vi "CRYSet Analysis Editor Front Panel.vi"(11 "Vi Ref":refnum<vi>) -> ()   [LabVIEW 2013]
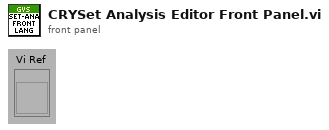
[diagram p1: front panel]
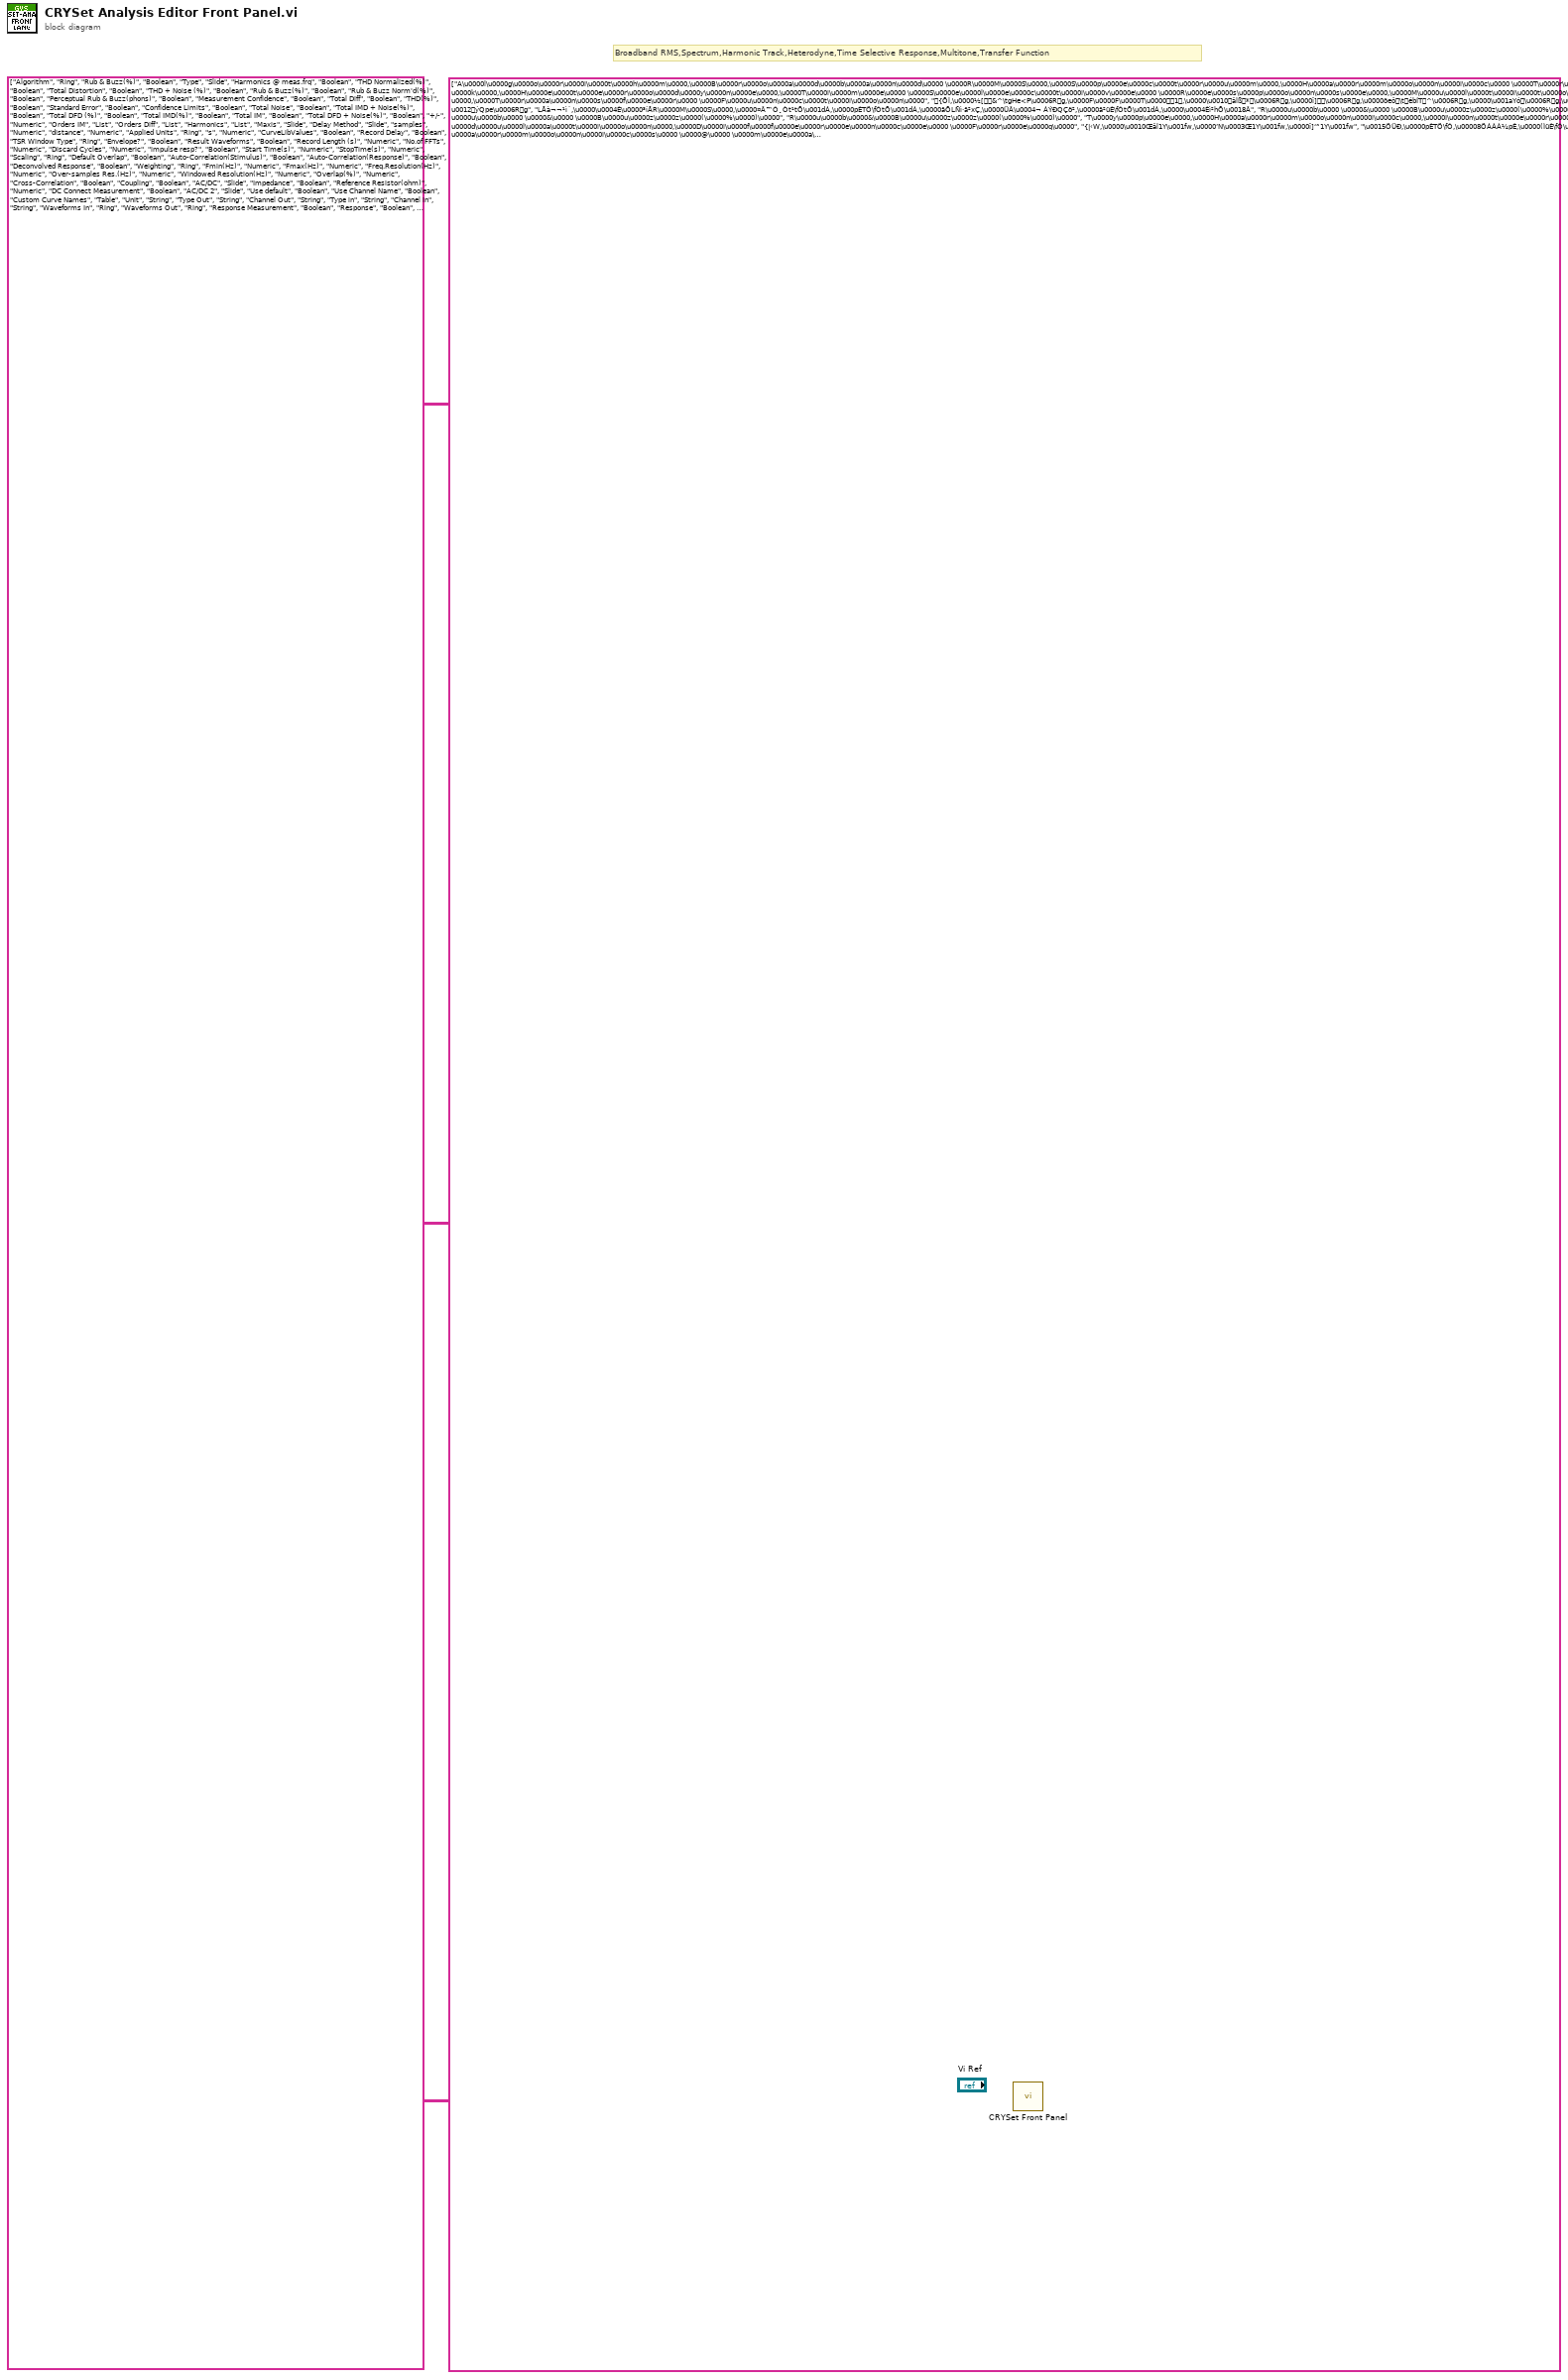
[diagram p0: block diagram]
diagram:
  # "Broadband RMS,Spectrum,Harmonic Track,Heterodyne,Time Selective Response,Multitone,Transfer Function"
  # "Caption, Tab Page, Multilist Header, Button 4"
  # "Control Type"
  # "Control Name and Tab"
  n1 = call "CRYSet Front Panel.vi"("Caption(Boolean Text)"=string[][] [["A\u0000l\u0000g\u0000o\u0000r\u0000i\u0000t\u0000h\u0000m\u0000,\u0000B\u0000r\u0000o\u0000a\u0000d\u0000b\u0000a\u0000n\u0000d\u0000 \u0000R\u0000M\u0000S\u0000,\u0000S\u0000p\u0000e\u0000c\u0000t\u0000r\u0000u\u0000m\u0000,\u0000H\u0000a\u0000r\u0000m\u0000o\u0000n\u0000i\u0000c\u0000 \u0000T\u0000r\u0000a\u0000c\u0000k\u0000,\u0000H\u0000e\u0000t\u0000e\u0000r\u0000o\u0000d\u0000y\u0000n\u0000e\u0000,\u0000T\u0000i\u0000m\u0000e\u0000 \u0000S\u0000e\u0000l\u0000e\u0000c\u0000t\u0000i\u0000v\u0000e\u0000 \u0000R\u0000e\u0000s\u0000p\u0000o\u0000n\u0000s\u0000e\u0000,\u0000M\u0000u\u0000l\u0000t\u0000i\u0000t\u0000o\u0000n\u0000e\u0000,\u0000T\u0000r\u0000a\u0000n\u0000s\u0000f\u0000e\u0000r\u0000 \u0000F\u0000u\u0000n\u0000c\u0000t\u0000i\u0000o\u0000n\u0000", "{Õl,\u0000½[&^\tgHe<P\u0006Rg,\u0000F\u0000F\u0000T\u00001,\u0000\u0010âlß*\u0006Rg,\u0000î]\u0006Rg,\u0000öeô\tébÍT^\u0006Rg,\u0000\u001aYó\u0006Rg,\u0000 O\u0012ýQpe\u0006Rg", "LÅà¬¬¹ì´,\u0000\u0004È\u0000³íÅR\u0000M\u0000S\u0000,\u0000¤Â™Ó¸Òt¹tÕ\u001dÁ,\u0000pÈTÖ\fÓtÕ\u001dÁ,\u0000äÕLÑì·ä²xÇ,\u0000ÜÂ\u0004¬ ÁÝÐQÇõ²,\u0000ä²üÈ\fÓtÕ\u001dÁ,\u0000\u0004Èì²hÕ\u0018Â"], ["R\u0000u\u0000b\u0000 \u0000&\u0000 \u0000B\u0000u\u0000z\u0000z\u0000(\u0000%\u0000)\u0000", "R\u0000u\u0000b\u0000 \u0000&\u0000 \u0000B\u0000u\u0000z\u0000z\u0000(\u0000%\u0000)\u0000", "R\u0000u\u0000b\u0000&\u0000B\u0000u\u0000z\u0000z\u0000(\u0000%\u0000)\u0000"], ["T\u0000y\u0000p\u0000e\u0000,\u0000H\u0000a\u0000r\u0000m\u0000o\u0000n\u0000i\u0000c\u0000,\u0000I\u0000n\u0000t\u0000e\u0000r\u0000m\u0000o\u0000d\u0000u\u0000l\u0000a\u0000t\u0000i\u0000o\u0000n\u0000,\u0000D\u0000i\u0000f\u0000f\u0000e\u0000r\u0000e\u0000n\u0000c\u0000e\u0000 \u0000F\u0000r\u0000e\u0000q\u0000", "{|‹W,\u0000\u0010Œâl1Y\u001fw,\u0000’N\u0003Œ1Y\u001fw,\u0000î]‘˜1Y\u001fw", "\u0015ÖÜÐ,\u0000pÈTÖ\fÓ,\u00008ÖÁÀÀ¼pÈ,\u0000(ÌüÈ\fÓ\u0018Â"], ["H\u0000a\u0000r\u0000m\u0000o\u0000n\u0000i\u0000c\u0000s\u0000 \u0000@\u0000 \u0000m\u0000e\u0000a\u0000s\u0000.\u0000f\u0000r\u0000q\u0000", "\u0010ŒâlKmÏ‘‘˜‡s", "pÈTÖ\fÓ!Î\u0015ÈüÈ\fÓ\u0018Â"], ["T\u0000H\u0000D\u0000 \u0000N\u0000o\u0000r\u0000m\u0000a\u0000l\u0000i\u0000z\u0000e\u0000d\u0000(\u0000%\u0000)\u0000", ";`\u0010Œâl1Y\u001fw(\u0000R_\u0000N\u0016S)\u0000(\u0000%\u0000)\u0000", "T\u0000H\u0000D\u0000\u0015ÈÜ­TÖ(\u0000%\u0000)\u0000"], ["T\u0000o\u0000t\u0000a\u0000l\u0000 \u0000D\u0000i\u0000s\u0000t\u0000o\u0000r\u0000t\u0000i\u0000o\u0000n\u0000", ";`1Y\u001fw", "\u0004È´ÌtÇÀÉì·ÐÉ"], ["T\u0000H\u0000D\u0000 \u0000+\u0000 \u0000N\u0000o\u0000i\u0000s\u0000e\u0000 \u0000(\u0000%\u0000)\u0000", ";`\u0010Œâl1Y\u001fw+\u0000jVðX(\u0000%\u0000)\u0000", "T\u0000H\u0000D\u0000+\u0000¡ÇLÇ(\u0000%\u0000)\u0000"], ["R\u0000u\u0000b\u0000 \u0000&\u0000 \u0000B\u0000u\u0000z\u0000z\u0000(\u0000%\u0000)\u0000", "\u0002_ó—", "R\u0000u\u0000b\u0000 \u0000&\u0000 \u0000B\u0000u\u0000z\u0000z\u0000(\u0000%\u0000)\u0000"], ["R\u0000u\u0000b\u0000 \u0000&\u0000 \u0000B\u0000u\u0000z\u0000z\u0000 \u0000N\u0000o\u0000r\u0000m\u0000'\u0000d\u0000(\u0000%\u0000)\u0000", "\u0002_ó—(\u0000R_\u0000N\u0016S)\u0000(\u0000%\u0000)\u0000", "R\u0000u\u0000b\u0000&\u0000B\u0000u\u0000z\u0000z\u0000\u0015ÈÜ­TÖ(\u0000%\u0000)\u0000"], ["P\u0000e\u0000r\u0000c\u0000e\u0000p\u0000t\u0000u\u0000a\u0000l\u0000 \u0000R\u0000u\u0000b\u0000 \u0000&\u0000 \u0000B\u0000u\u0000z\u0000z\u0000(\u0000p\u0000h\u0000o\u0000n\u0000s\u0000)\u0000", "\u001faåw\u0002_ó—(\u0000p\u0000h\u0000o\u0000n\u0000s\u0000)\u0000", "ÀÉ\u0001¬ \u0000R\u0000u\u0000b\u0000 \u0000&\u0000 \u0000B\u0000u\u0000z\u0000z\u0000(\u0000p\u0000h\u0000o\u0000n\u0000s\u0000)\u0000"], ["M\u0000e\u0000a\u0000s\u0000u\u0000r\u0000e\u0000m\u0000e\u0000n\u0000t\u0000 \u0000C\u0000o\u0000n\u0000f\u0000i\u0000d\u0000e\u0000n\u0000c\u0000e\u0000", "KmÏ‘náO¦^", "ÿ»LÇ1Á!Î\u0015È"], ["T\u0000o\u0000t\u0000a\u0000l\u0000 \u0000D\u0000i\u0000f\u0000f\u0000", ";`î]\u0002_", "\u0004È´Ì \u0000(ÌtÇÀÉì·ÐÉ"], ["T\u0000H\u0000D\u0000(\u0000%\u0000)\u0000", ";`\u0010Œâl1Y\u001fw(\u0000%\u0000)\u0000", "T\u0000H\u0000D\u0000(\u0000%\u0000)\u0000"], ["S\u0000t\u0000a\u0000n\u0000d\u0000a\u0000r\u0000d\u0000 \u0000E\u0000r\u0000r\u0000o\u0000r\u0000", "\u0007hÆQî]", "\\Ô\u0000É$Æ(Ì"], ["C\u0000o\u0000n\u0000f\u0000i\u0000d\u0000e\u0000n\u0000c\u0000e\u0000 \u0000L\u0000i\u0000m\u0000i\u0000t\u0000s\u0000", "náOLuP–", "ÿ»LÇ1Á\\ÕÄ¬"], ["T\u0000o\u0000t\u0000a\u0000l\u0000 \u0000N\u0000o\u0000i\u0000s\u0000e\u0000", ";`jVðX", "\u0004È´Ì¡ÇLÇ"], ["T\u0000o\u0000t\u0000a\u0000l\u0000 \u0000I\u0000M\u0000D\u0000 \u0000+\u0000 \u0000N\u0000o\u0000i\u0000s\u0000e\u0000(\u0000%\u0000)\u0000", "qQ\tgI\u0000M\u0000D\u0000+\u0000jVðX(\u0000%\u0000)\u0000", "\u0004È´Ì \u0000I\u0000M\u0000D\u0000+\u0000¡ÇLÇ(\u0000%\u0000)\u0000"], ["T\u0000o\u0000t\u0000a\u0000l\u0000 \u0000D\u0000F\u0000D\u0000 \u0000(\u0000%\u0000)\u0000", "qQ\tgD\u0000F\u0000D\u0000(\u0000%\u0000)\u0000", "\u0004È´Ì \u0000D\u0000F\u0000D\u0000 \u0000(\u0000%\u0000)\u0000"], ["T\u0000o\u0000t\u0000a\u0000l\u0000 \u0000I\u0000M\u0000D\u0000(\u0000%\u0000)\u0000", "qQ\tgI\u0000M\u0000D\u0000(\u0000%\u0000)\u0000", "\u0004È´Ì \u0000I\u0000M\u0000D\u0000(\u0000%\u0000)\u0000"], ["T\u0000o\u0000t\u0000a\u0000l\u0000 \u0000I\u0000M\u0000", "qQ\tgI\u0000M\u0000", "\u0004È´Ì \u0000I\u0000M\u0000tÇÀÉì·ÐÉ"], ["T\u0000o\u0000t\u0000a\u0000l\u0000 \u0000D\u0000F\u0000D\u0000 \u0000+\u0000 \u0000N\u0000o\u0000i\u0000s\u0000e\u0000(\u0000%\u0000)\u0000", "qQ\tgD\u0000F\u0000D\u0000+\u0000jVðX(\u0000%\u0000)\u0000", "\u0004È´Ì \u0000D\u0000F\u0000D\u0000+\u0000¡ÇLÇ(\u0000%\u0000)\u0000"], ["S\u0000t\u0000d\u0000 \u0000E\u0000r\u0000r\u0000", "\u0007hÆQ\u0019•ï‹", "\\Ô\u0000É$Æ(Ì"], ["O\u0000r\u0000d\u0000e\u0000r\u0000s\u0000", "!kpe", "(Ì\u0018Â"], ["O\u0000r\u0000d\u0000e\u0000r\u0000s\u0000", "!kpe", "(Ì\u0018Â"], ["H\u0000a\u0000r\u0000m\u0000o\u0000n\u0000i\u0000c\u0000s\u0000", "\u0010Œâl", "pÈTÖ\fÓ"], ["M\u0000a\u0000x\u0000i\u0000s\u0000,\u0000x\u0000,\u0000y\u0000,\u0000z\u0000", "t,\u0000x\u0000,\u0000y\u0000,\u0000z\u0000", "Ç¬¹\\ÔÍ,\u0000x\u0000,\u0000y\u0000,\u0000z\u0000"], ["D\u0000e\u0000l\u0000a\u0000y\u0000 \u0000M\u0000e\u0000t\u0000h\u0000o\u0000d\u0000,\u0000A\u0000u\u0000t\u0000o\u0000 \u0000D\u0000e\u0000l\u0000a\u0000y\u0000,\u0000S\u0000e\u0000t\u0000 \u0000V\u0000a\u0000l\u0000u\u0000e\u0000s\u0000,\u0000C\u0000u\u0000r\u0000v\u0000e\u0000s\u0000 \u0000L\u0000i\u0000b\u0000r\u0000a\u0000r\u0000y\u0000", "ö^ß¹eÕl,\u0000ê¨Rö^öe,\u0000¾[<P,\u0000òf¿~^", "ÀÉðÅ)¼¼,\u0000ÇÙ³ÀÉðÅ,\u0000\u0012¬$Á\u0015È,\u0000á¬ Á\u001cÁà¬¬¹©Æ"], ["s\u0000a\u0000m\u0000p\u0000l\u0000e\u0000s\u0000", "7h,g", "\\Ôø¼\u001c¬\u0018Â"], ["d\u0000i\u0000s\u0000t\u0000a\u0000n\u0000c\u0000e\u0000", "Ý»y", "p¬¬¹"], ["A\u0000p\u0000p\u0000l\u0000i\u0000e\u0000d\u0000 \u0000U\u0000n\u0000i\u0000t\u0000s\u0000", "”^(uUSMO", "\u0001È©Æè²\u0004Ç"], ["s\u0000", "Òy", "\bÍ"], ["C\u0000u\u0000r\u0000v\u0000e\u0000L\u0000i\u0000b\u0000r\u0000a\u0000r\u0000y\u0000V\u0000a\u0000l\u0000u\u0000e\u0000s\u0000", "òf¿~<P", "á¬ Á\u001cÁà¬\u0012¬"], ["R\u0000e\u0000c\u0000o\u0000r\u0000d\u0000 \u0000D\u0000e\u0000l\u0000a\u0000y\u0000", "°U_ö^ß", "0®]¸ÀÉðÅ"], ["T\u0000S\u0000R\u0000 \u0000W\u0000i\u0000n\u0000d\u0000o\u0000w\u0000 \u0000T\u0000y\u0000p\u0000e\u0000", "T\u0000S\u0000R\u0000—zýQpe{|‹W", "T\u0000S\u0000R\u0000=ÌhÕ\u0018Â"], ["T\u0000i\u0000m\u0000e\u0000 \u0000E\u0000n\u0000v\u0000e\u0000l\u0000o\u0000p\u0000e\u0000", "öeô•\u0005SÜ~", "ÜÂ\u0004¬ìÓ}·"], ["R\u0000e\u0000s\u0000u\u0000l\u0000t\u0000 \u0000W\u0000a\u0000v\u0000e\u0000f\u0000o\u0000r\u0000m\u0000s\u0000", "Ó~œgâlb_", "°¬ü¬\fÓ\u0015Ö"], ["R\u0000e\u0000c\u0000o\u0000r\u0000d\u0000 \u0000L\u0000e\u0000n\u0000g\u0000t\u0000h\u0000 \u0000(\u0000s\u0000)\u0000", "F\u0000F\u0000T\u0000•¦^(\u0000s\u0000)\u0000", "0®]¸8®tÇ(\u0000\bÍ)\u0000"], ["N\u0000o\u0000.\u0000o\u0000f\u0000 \u0000F\u0000F\u0000T\u0000s\u0000", "F\u0000F\u0000T\u0000peϑ", "F\u0000F\u0000T\u0000\u0014¾\\¸lÐ\u001c¬\u0018Â"], ["D\u0000i\u0000s\u0000c\u0000a\u0000r\u0000d\u0000 \u0000C\u0000y\u0000c\u0000l\u0000e\u0000s\u0000", "\"N\u0003_hT\u001fg", "„¼¼¹üÈ0®"], ["I\u0000m\u0000p\u0000u\u0000l\u0000s\u0000e\u0000 \u0000R\u0000e\u0000s\u0000p\u0000.\u0000", "²QûQÍT”^", "„Ç\fÕ¤ÂQÇõ²"], ["S\u0000t\u0000a\u0000r\u0000t\u0000 \u0000T\u0000i\u0000m\u0000e\u0000(\u0000s\u0000)\u0000", "\u0000_ËYöeô•(\u0000Òy)\u0000", "ÜÂ‘ÇÜÂ\u0004¬(\u0000\bÍ)\u0000"], ["S\u0000t\u0000o\u0000p\u0000 \u0000T\u0000i\u0000m\u0000e\u0000(\u0000s\u0000)\u0000", "\\Pbköeô•(\u0000Òy)\u0000", "\u0015ÈÀÉÜÂ\u0004¬(\u0000\bÍ)\u0000"], ["S\u0000c\u0000a\u0000l\u0000i\u0000n\u0000g\u0000", ";R¦^", "™ÌÄ³"], ["D\u0000e\u0000f\u0000a\u0000u\u0000l\u0000t\u0000 \u0000O\u0000v\u0000e\u0000r\u0000l\u0000a\u0000p\u0000", "Øž¤‹Í‘àS", "0®\u0015È¹¬hÎ"], ["A\u0000u\u0000t\u0000o\u0000-\u0000C\u0000o\u0000r\u0000r\u0000e\u0000l\u0000a\u0000t\u0000i\u0000o\u0000n\u0000(\u0000S\u0000t\u0000i\u0000m\u0000u\u0000l\u0000u\u0000s\u0000)\u0000", "ê¨RøvsQ(\u0000Ào±R)\u0000", "ÇÙ³ÁÀ\u0000­(\u0000Çù­)\u0000"], ["A\u0000u\u0000t\u0000o\u0000-\u0000C\u0000o\u0000r\u0000r\u0000e\u0000l\u0000a\u0000t\u0000i\u0000o\u0000n\u0000(\u0000R\u0000e\u0000s\u0000p\u0000o\u0000n\u0000s\u0000e\u0000)\u0000", "ê¨RøvsQ(\u0000ÍT^)\u0000", "ÇÙ³ÁÀ\u0000­(\u0000QÇõ²)\u0000"], ["D\u0000e\u0000c\u0000o\u0000n\u0000v\u0000o\u0000l\u0000v\u0000e\u0000d\u0000 \u0000R\u0000e\u0000s\u0000p\u0000o\u0000n\u0000s\u0000e\u0000", "\u0006wSïyÍT^", "íÅ\u0011É©ÌQÇõ²"], ["W\u0000e\u0000i\u0000g\u0000h\u0000t\u0000i\u0000n\u0000g\u0000", " RCg", "4»Œ¬"], ["F\u0000m\u0000i\u0000n\u0000(\u0000H\u0000z\u0000)\u0000", "\u0000gNO‘˜‡s(\u0000H\u0000z\u0000)\u0000", "\\ÍŒÁüÈ\fÓ\u0018Â(\u0000H\u0000z\u0000)\u0000"], ["F\u0000m\u0000a\u0000x\u0000(\u0000H\u0000z\u0000)\u0000", "\u0000g'Y‘˜‡s(\u0000H\u0000z\u0000)\u0000", "\\Í\u0000³üÈ\fÓ\u0018Â(\u0000H\u0000z\u0000)\u0000"], ["F\u0000r\u0000e\u0000q\u0000.\u0000R\u0000e\u0000s\u0000o\u0000l\u0000u\u0000t\u0000i\u0000o\u0000n\u0000(\u0000H\u0000z\u0000)\u0000", "‘˜‡sÍT”^(\u0000H\u0000z\u0000)\u0000", "üÈ\fÓ\u0018Â„½tÕ¥²(\u0000H\u0000z\u0000)\u0000"], ["O\u0000v\u0000e\u0000r\u0000-\u0000s\u0000a\u0000m\u0000p\u0000l\u0000e\u0000s\u0000 \u0000R\u0000e\u0000s\u0000.\u0000(\u0000H\u0000z\u0000)\u0000", "òf¿~\u0006R¨s(\u0000H\u0000z\u0000)\u0000", "\u0004È´Ì\\Ôø¼„½tÕ¥²(\u0000H\u0000z\u0000)\u0000"], ["W\u0000i\u0000n\u0000d\u0000o\u0000w\u0000e\u0000d\u0000 \u0000R\u0000e\u0000s\u0000o\u0000l\u0000u\u0000t\u0000i\u0000o\u0000n\u0000(\u0000H\u0000z\u0000)\u0000", "zýQpe\u0006R¨s(\u0000H\u0000z\u0000)\u0000", "=Ì„½tÕ¥²(\u0000H\u0000z\u0000)\u0000"], ["O\u0000v\u0000e\u0000r\u0000l\u0000a\u0000p\u0000(\u0000%\u0000)\u0000", "Í‘àS(\u0000%\u0000)\u0000", "¹¬hÎ(\u0000%\u0000)\u0000"], ["C\u0000r\u0000o\u0000s\u0000s\u0000-\u0000C\u0000o\u0000r\u0000r\u0000e\u0000l\u0000a\u0000t\u0000i\u0000o\u0000n\u0000", "’NøvsQ", "8ÖÁÀÁÀ\u0000­"], ["C\u0000o\u0000u\u0000p\u0000l\u0000i\u0000n\u0000g\u0000", "&€\bT", "°¬iÕ"], ["A\u0000C\u0000/\u0000D\u0000C\u0000,\u0000A\u0000C\u0000,\u0000D\u0000C\u0000", "A\u0000C\u0000/\u0000D\u0000C\u0000,\u0000¤NAm,\u0000ôvAm", "P­X¹/\u0000ÁÉX¹,\u0000P­X¹,\u0000ÁÉX¹"], ["I\u0000m\u0000p\u0000e\u0000d\u0000a\u0000n\u0000c\u0000e\u0000", ";–—b", "DÆ\u0004È\u0000ÈmÕ"], ["R\u0000e\u0000f\u0000e\u0000r\u0000e\u0000n\u0000c\u0000e\u0000 \u0000R\u0000e\u0000s\u0000i\u0000s\u0000t\u0000o\u0000r\u0000(\u0000o\u0000h\u0000m\u0000)\u0000", "ÂS\u0003€5u;–(\u0000o\u0000h\u0000m\u0000)\u0000", "8Ìà¬\u0000ÈmÕ(\u0000o\u0000h\u0000m\u0000)\u0000"], ["D\u0000C\u0000 \u0000C\u0000o\u0000n\u0000n\u0000e\u0000c\u0000t\u0000 \u0000M\u0000e\u0000a\u0000s\u0000u\u0000r\u0000e\u0000m\u0000e\u0000n\u0000t\u0000", "D\u0000C\u0000Þ¥cKmÏ", "ÁÉX¹(¸°¬!Î\u0015È"], ["A\u0000C\u0000/\u0000D\u0000C\u0000 \u00002\u0000,\u0000A\u0000(\u0000 \u0000i\u0000n\u0000 \u0000V\u0000o\u0000l\u0000t\u0000a\u0000g\u0000e\u0000 \u0000s\u0000o\u0000u\u0000r\u0000c\u0000e\u0000 \u0000M\u0000o\u0000d\u0000e\u0000)\u0000,\u0000V\u0000(\u0000 \u0000i\u0000n\u0000 \u0000C\u0000u\u0000r\u0000r\u0000e\u0000n\u0000t\u0000 \u0000s\u0000o\u0000u\u0000r\u0000c\u0000e\u0000 \u0000M\u0000o\u0000d\u0000e\u0000)\u0000", "A\u0000C\u0000/\u0000D\u0000C\u0000 \u00002\u0000,\u0000A\u0000(\u00005uSn!j\u000f_)\u0000,\u0000V\u0000(\u0000(W5uAmn!j\u000f_)\u0000", "P­X¹/\u0000ÁÉX¹,\u0000TÅ˜ÓDÅ(\u0000\u0004ÈUÅÐÆœÌ)¼ÝÂ)\u0000,\u0000ü¼¸Ò(\u0000\u0004ÈX¹ÐÆœÌ)¼ÝÂ)\u0000"], ["U\u0000s\u0000e\u0000 \u0000d\u0000e\u0000f\u0000a\u0000u\u0000l\u0000t\u0000", "O(uØž¤‹", "0®\u0015È¬À©Æ"], ["U\u0000s\u0000e\u0000 \u0000C\u0000h\u0000a\u0000n\u0000n\u0000e\u0000l\u0000 \u0000N\u0000a\u0000m\u0000e\u0000", "O(uS\rTðy", "µÑ\\¸tÇ„¹¬À©Æ"], ["C\u0000u\u0000s\u0000t\u0000o\u0000m\u0000 \u0000C\u0000u\u0000r\u0000v\u0000e\u0000 \u0000N\u0000a\u0000m\u0000e\u0000s\u0000", "ê[INvòf¿~\rTðy", "á¬ ÁtÇ„¹\u0015ÈXÇ"], ["U\u0000n\u0000i\u0000t\u0000", "USMO", "è²\u0004Ç"], ["T\u0000y\u0000p\u0000e\u0000 \u0000O\u0000u\u0000t\u0000", "úQ{|W", "œÍl­\u0015ÖÜÐ"], ["C\u0000h\u0000a\u0000n\u0000n\u0000e\u0000l\u0000 \u0000O\u0000u\u0000t\u0000", "úQ\u001aS", "œÍl­µÑ\\¸"], ["T\u0000y\u0000p\u0000e\u0000 \u0000i\u0000n\u0000", "eQ{|W", "…Çl­\u0015ÖÜÐ"], ["C\u0000h\u0000a\u0000n\u0000n\u0000e\u0000l\u0000 \u0000i\u0000n\u0000", "eQ\u001aS", "…Çl­µÑ\\¸"], ["W\u0000a\u0000v\u0000e\u0000f\u0000o\u0000r\u0000m\u0000s\u0000 \u0000I\u0000n\u0000", "eQâlb_", "…Çl­\fÓ\u0015Ö"], ["W\u0000a\u0000v\u0000e\u0000f\u0000o\u0000r\u0000m\u0000s\u0000 \u0000O\u0000u\u0000t\u0000", "úQâlb_", "œÍl­\fÓ\u0015Ö"], ["R\u0000e\u0000s\u0000p\u0000o\u0000n\u0000s\u0000e\u0000 \u0000M\u0000e\u0000a\u0000s\u0000u\u0000r\u0000e\u0000m\u0000e\u0000n\u0000t\u0000", "ÍT”^KmÏ‘", "QÇõ²!Î\u0015È"], ["R\u0000e\u0000s\u0000p\u0000o\u0000n\u0000s\u0000e\u0000", "ÍT”^", "QÇõ²"], ["S\u0000t\u0000i\u0000m\u0000u\u0000l\u0000u\u0000s\u0000", "Ào±R", "Çù­"], ["R\u0000e\u0000s\u0000p\u0000o\u0000n\u0000s\u0000e\u0000 \u0000M\u0000e\u0000a\u0000s\u0000u\u0000r\u0000e\u0000m\u0000e\u0000n\u0000t\u00001\u0000,\u0000A\u0000b\u0000s\u0000o\u0000l\u0000u\u0000t\u0000e\u0000,\u0000R\u0000e\u0000l\u0000a\u0000t\u0000i\u0000v\u0000e\u0000", "‘˜ÍTKmÏ‘<P,\u0000Ý~ù[<P,\u0000øvù[<P", "QÇõ²!Î\u0015È,\u0000\bÈ\u0000³,\u0000ÁÀ\u0000³"], ["A\u0000p\u0000p\u0000l\u0000y\u0000 \u0000C\u0000o\u0000r\u0000r\u0000e\u0000c\u0000t\u0000i\u0000o\u0000n\u0000 \u0000O\u0000u\u0000t\u0000", "^(uúQîOck", "œÍl­ô¼\u0015È\u0001È©Æ"], ["A\u0000p\u0000p\u0000l\u0000y\u0000 \u0000C\u0000o\u0000r\u0000r\u0000e\u0000c\u0000t\u0000i\u0000o\u0000n\u0000 \u0000i\u0000n\u0000", "^(ueQîOck", "…Çl­ô¼\u0015È\u0001È©Æ"], ["A\u0000v\u0000e\u0000r\u0000a\u0000g\u0000i\u0000n\u0000g\u0000", "s^GW", "ÉÓà­"], ["F\u0000u\u0000n\u0000c\u0000t\u0000i\u0000o\u0000n\u0000s\u0000", "ŸRý€", "0®¥²"], ["S\u0000p\u0000e\u0000c\u0000t\u0000r\u0000a\u0000l\u0000 \u0000S\u0000c\u0000a\u0000l\u0000i\u0000n\u0000g\u0000*\u0000,\u0000R\u0000M\u0000S\u0000,\u0000S\u0000p\u0000e\u0000c\u0000t\u0000r\u0000a\u0000l\u0000 \u0000D\u0000e\u0000n\u0000s\u0000i\u0000t\u0000y\u0000", "‘˜1Œ)>e*\u0000,\u0000\tgHe<P,\u0000‘˜1ŒÆ[¦^", "¤Â™Ó¸Òt¹™ÌÄ³,\u0000R\u0000M\u0000S\u0000,\u0000S\u0000p\u0000e\u0000c\u0000t\u0000r\u0000a\u0000l\u0000 \u0000D\u0000e\u0000n\u0000s\u0000i\u0000t\u0000y\u0000"], ["A\u0000u\u0000t\u0000o\u0000-\u0000S\u0000p\u0000e\u0000c\u0000t\u0000r\u0000u\u0000m\u0000(\u0000S\u0000t\u0000i\u0000m\u0000u\u0000l\u0000u\u0000s\u0000)\u0000*\u0000", "ê¨R1(\u0000Ào±R)\u0000", "ÇÙ³¤ÂÓ¸Òt¹(\u0000Çù­)\u0000"], ["A\u0000u\u0000t\u0000o\u0000-\u0000S\u0000p\u0000e\u0000c\u0000t\u0000r\u0000u\u0000m\u0000(\u0000R\u0000e\u0000s\u0000p\u0000o\u0000n\u0000s\u0000e\u0000)\u0000*\u0000", "ê¨R1(\u0000ÍT^)\u0000", "ÇÙ³¤ÂÓ¸Òt¹(\u0000QÇõ²)\u0000"], ["C\u0000r\u0000o\u0000s\u0000s\u0000-\u0000S\u0000p\u0000e\u0000c\u0000t\u0000r\u0000u\u0000m\u0000*\u0000", "¤NÉS‘˜1Œ*\u0000", "P­(Ì¤Â™Ó¸Òt¹"], ["C\u0000o\u0000h\u0000e\u0000r\u0000e\u0000n\u0000t\u0000 \u0000P\u0000o\u0000w\u0000e\u0000r\u0000*\u0000", "øvr^ŸR‡s*\u0000", "\u0004¬-Á\u0004È%¸"], ["F\u0000r\u0000e\u0000q\u0000u\u0000e\u0000n\u0000c\u0000y\u0000 \u0000R\u0000e\u0000s\u0000p\u0000o\u0000n\u0000s\u0000e\u0000", "‘˜‡sÍT”^", "üÈ\fÓ\u0018ÂQÇõ²"], ["N\u0000o\u0000n\u0000-\u0000C\u0000o\u0000h\u0000e\u0000r\u0000e\u0000n\u0000t\u0000 \u0000P\u0000o\u0000w\u0000e\u0000r\u0000*\u0000", "^—øvr^ŸR‡s*\u0000", "D¾\u0004¬-Á\u0004È%¸"], ["C\u0000o\u0000h\u0000e\u0000r\u0000e\u0000n\u0000c\u0000e\u0000 \u0000(\u0000%\u0000)\u0000", "øvr^(\u0000%\u0000)\u0000", "\u0004¬-Á1Á(\u0000%\u0000)\u0000"], ["N\u0000o\u0000n\u0000-\u0000C\u0000o\u0000h\u0000e\u0000r\u0000e\u0000n\u0000c\u0000e\u0000 \u0000(\u0000%\u0000)\u0000", "^—øvr^(\u0000%\u0000)\u0000", "D¾\u0004¬-Á1Á(\u0000%\u0000)\u0000"], ["S\u0000i\u0000g\u0000n\u0000a\u0000l\u0000-\u0000N\u0000o\u0000i\u0000s\u0000e\u0000 \u0000R\u0000a\u0000t\u0000i\u0000o\u0000 \u0000(\u0000d\u0000B\u0000)\u0000", "áOjVÔk(\u0000d\u0000B\u0000)\u0000", "àÂ8Ö\u0000³¡ÇLÇD¾(\u0000%\u0000)\u0000"], ["N\u0000o\u0000n\u0000-\u0000C\u0000o\u0000h\u0000e\u0000r\u0000e\u0000n\u0000t\u0000 \u0000D\u0000i\u0000s\u0000t\u0000o\u0000r\u0000t\u0000i\u0000o\u0000n\u0000*\u0000", "^—øvr^1Y\u001fw", "D¾\u0004¬-ÁtÇÀÉì·ÐÉ"], ["A\u0000v\u0000e\u0000r\u0000a\u0000g\u0000i\u0000n\u0000g\u00001\u0000,\u0000C\u0000o\u0000m\u0000p\u0000l\u0000e\u0000x\u0000,\u0000P\u0000o\u0000w\u0000e\u0000r\u0000", "s^GW,\u0000\rY\bT,\u0000ŸR‡s", "ÉÓà­,\u0000õ¼ŒÁ,\u0000\u0004È%¸"], ["L\u0000o\u0000o\u0000s\u0000e\u0000 \u0000P\u0000a\u0000r\u0000t\u0000i\u0000c\u0000l\u0000e\u0000", "~gce»yP[", "Ç Ç½¹Ç"], ["L\u0000o\u0000o\u0000s\u0000e\u0000 \u0000P\u0000a\u0000r\u0000t\u0000i\u0000c\u0000l\u0000e\u0000 \u0000W\u0000a\u0000v\u0000e\u0000f\u0000o\u0000r\u0000m\u0000", "~gce»yP[âlb_", "Ç Ç½¹Ç\fÓ\u0015Ö"], ["A\u0000v\u0000e\u0000r\u0000a\u0000g\u0000i\u0000n\u0000g\u0000 \u0000T\u0000i\u0000m\u0000e\u0000(\u0000s\u0000)\u0000", "s^GWöeô•(\u0000s\u0000)\u0000", "ÉÓà­ÜÂ\u0004¬(\u0000\bÍ)\u0000"], ["A\u0000t\u0000t\u0000a\u0000c\u0000k\u0000 \u0000T\u0000h\u0000r\u0000e\u0000s\u0000h\u0000o\u0000l\u0000d\u0000(\u0000d\u0000B\u0000)\u0000", "ÀoÑSLuP–(\u0000d\u0000B\u0000)\u0000", "õ¬©¬1Ñ\u0012¬(\u0000d\u0000B\u0000)\u0000"], ["M\u0000a\u0000x\u0000 \u0000d\u0000u\u0000r\u0000a\u0000t\u0000i\u0000o\u0000n\u0000(\u0000s\u0000)\u0000", "\u0000g'Y\u0001cí~öeô•(\u0000s\u0000)\u0000", "\\Í\u0000³ÀÉÁÜÂ\u0004¬(\u0000\bÍ)\u0000"], ["M\u0000i\u0000n\u0000 \u0000d\u0000u\u0000r\u0000a\u0000t\u0000i\u0000o\u0000n\u0000(\u0000s\u0000)\u0000", "\u0000g\u000f\\\u0001cí~öeô•(\u0000s\u0000)\u0000", "\\ÍÁÀÉÁÜÂ\u0004¬(\u0000\bÍ)\u0000"], ["H\u0000y\u0000s\u0000t\u0000e\u0000r\u0000e\u0000s\u0000i\u0000s\u0000 \u0000U\u0000p\u0000(\u0000d\u0000B\u0000)\u0000", "ÁxÞn°saŒ\nNGS(\u0000d\u0000B\u0000)\u0000", "ÃÆÇ0®¬¹%¸(\u0000d\u0000B\u0000)\u0000"], ["A\u0000p\u0000p\u0000l\u0000y\u0000", "”^(u", "\u0001È©Æ"], ["U\u0000n\u0000i\u0000t\u0000s\u0000.\u0000.\u0000.\u0000", "USMO", "è²\u0004Ç$Á\u0015È"], ["E\u0000d\u0000i\u0000t\u0000 \u0000L\u0000i\u0000s\u0000t\u0000", "\u0016\u0017Rh", "¸ÓÑÉ©º]¸"], ["C\u0000u\u0000r\u0000v\u0000e\u0000s\u0000,\u0000D\u0000e\u0000l\u0000a\u0000y\u0000,\u0000F\u0000r\u0000e\u0000q\u0000u\u0000e\u0000n\u0000c\u0000y\u0000,\u0000L\u0000o\u0000o\u0000s\u0000e\u0000 \u0000P\u0000a\u0000r\u0000t\u0000,\u0000W\u0000a\u0000v\u0000e\u0000f\u0000o\u0000r\u0000m\u0000s\u0000,\u0000D\u0000i\u0000s\u0000t\u0000o\u0000r\u0000t\u0000i\u0000o\u0000n\u0000,\u0000T\u0000i\u0000m\u0000e\u0000,\u0000E\u0000e\u0000l\u0000e\u0000c\u0000t\u0000r\u0000i\u0000c\u0000a\u0000l\u0000,\u0000H\u0000e\u0000l\u0000p\u0000", "òf¿~,\u0000ö^ß,\u0000s,\u0000~gce»yP[,\u0000âlb_,\u00001Y\u001fw,\u0000öeô,\u00005uáO÷S,\u0000.^©R", "Íl­á¬ Á,\u0000ÀÉðÅ,\u0000üÈ\fÓ\u0018Â,\u0000Ç Ç½¹Ç,\u0000ÜÂ\u0004¬\fÓ\u0015Ö,\u0000tÇÀÉì·ÐÉ,\u0000ÜÂ\u0004¬,\u0000\u0004È0®,\u0000Ä³ÀÆÐ¹"], ["A\u0000d\u0000v\u0000a\u0000n\u0000c\u0000e\u0000d\u0000 \u0000V\u0000i\u0000e\u0000w\u0000", "Ø§~\ty", "Ç8Á× \u0000ô¼0®"], ["M\u0000e\u0000t\u0000h\u0000o\u0000d\u0000,\u0000I\u0000E\u0000C\u0000 \u0000M\u0000e\u0000t\u0000h\u0000o\u0000d\u0000,\u0000I\u0000E\u0000E\u0000E\u0000 \u0000M\u0000e\u0000t\u0000h\u0000o\u0000d\u0000", "¹eÕl,\u0000I\u0000E\u0000C\u0000¹eÕl,\u0000I\u0000E\u0000E\u0000E\u0000¹eÕl", ")¼•¼,\u0000I\u0000E\u0000C\u0000 \u0000)¼•¼,\u0000I\u0000E\u0000E\u0000E\u0000 \u0000)¼•¼"], ["I\u0000m\u0000p\u0000e\u0000d\u0000a\u0000n\u0000c\u0000e\u0000", ";–—b", "DÆ\u0004È\u0000ÈmÕ"], ["S\u0000p\u0000e\u0000c\u0000t\u0000r\u0000a\u0000", "‘˜1Œ", "¤Â™Ó¸Òt¹"], ["D\u0000i\u0000s\u0000t\u0000a\u0000n\u0000c\u0000e\u0000 \u0000U\u0000n\u0000i\u0000t\u0000,\u0000i\u0000n\u0000c\u0000h\u0000e\u0000s\u0000,\u0000m\u0000e\u0000t\u0000e\u0000r\u0000s\u0000", "Ý»yUSMO,\u0000ñø[,\u0000s|", "D\u0000i\u0000s\u0000t\u0000a\u0000n\u0000c\u0000e\u0000 \u0000U\u0000n\u0000i\u0000t\u0000,\u0000i\u0000n\u0000c\u0000h\u0000e\u0000s\u0000,\u0000m\u0000e\u0000t\u0000e\u0000r\u0000s\u0000"], ["C\u0000u\u0000r\u0000v\u0000e\u0000 \u0000R\u0000e\u0000s\u0000o\u0000l\u0000u\u0000t\u0000i\u0000o\u0000n\u0000", "òf¿~\u0006R¨", "á¬ Á„½tÕ¥²"], ["P\u0000o\u0000l\u0000a\u0000r\u0000i\u0000t\u0000y\u0000", "g'`", "ù­1Á"], ["I\u0000m\u0000p\u0000e\u0000d\u0000a\u0000n\u0000c\u0000e\u0000", ";–—b", "„Ç<ÕX³¤Â"], ["A\u0000m\u0000p\u0000 \u0000A\u0000u\u0000t\u0000o\u0000 \u0000M\u0000o\u0000d\u0000e\u0000,\u0000A\u0000u\u0000t\u0000o\u0000m\u0000a\u0000t\u0000i\u0000c\u0000,\u0000M\u0000a\u0000n\u0000u\u0000a\u0000l\u0000", "L\u0000a\u0000n\u0000g\u0000u\u0000a\u0000g\u0000e\u0000 \u0000M\u0000o\u0000d\u0000e\u0000,\u0000ê¨R,\u0000Kb¨R", "L\u0000a\u0000n\u0000g\u0000u\u0000a\u0000g\u0000e\u0000 \u0000M\u0000o\u0000d\u0000e\u0000,\u0000ÇÙ³,\u0000\u0018ÂÙ³"], ["M\u0000i\u0000c\u0000r\u0000o\u0000p\u0000h\u0000o\u0000n\u0000e\u0000", "¦žKQÎ˜", "È¹tÇlÐ"], ["M\u0000i\u0000c\u0000 \u0000R\u0000e\u0000s\u0000i\u0000s\u0000t\u0000o\u0000r\u0000(\u0000o\u0000h\u0000m\u0000)\u0000", "¦žKQÎ˜5u;–(\u0000o\u0000h\u0000m\u0000)\u0000", "È¹tÇlÐ\u0000ÈmÕ(\u0000o\u0000h\u0000m\u0000)\u0000"], ["A\u0000m\u0000p\u0000 \u0000A\u0000u\u0000t\u0000o\u0000 \u0000M\u0000o\u0000d\u0000e\u0000,\u0000A\u0000u\u0000t\u0000o\u0000m\u0000a\u0000t\u0000i\u0000c\u0000,\u0000M\u0000a\u0000n\u0000u\u0000a\u0000l\u0000", "L\u0000a\u0000n\u0000g\u0000u\u0000a\u0000g\u0000e\u0000 \u0000M\u0000o\u0000d\u0000e\u0000,\u0000ê¨R,\u0000Kb¨R", "L\u0000a\u0000n\u0000g\u0000u\u0000a\u0000g\u0000e\u0000 \u0000M\u0000o\u0000d\u0000e\u0000,\u0000ÇÙ³,\u0000\u0018ÂÙ³"], ["M\u0000i\u0000c\u0000 \u0000C\u0000u\u0000r\u0000r\u0000e\u0000n\u0000t\u0000", "¦žKQÎ˜5uAm", "È¹tÇlÐ\u0004ÈX¹"]], "Control ID and Type(Label Name, Type)"=string[][] [["Algorithm", "Ring"], ["Rub & Buzz(%)", "Boolean"], ["Type", "Slide"], ["Harmonics @ meas.frq", "Boolean"], ["THD Normalized(%)", "Boolean"], ["Total Distortion", "Boolean"], ["THD + Noise (%)", "Boolean"], ["Rub & Buzz(%)", "Boolean"], ["Rub & Buzz Norm'd(%)", "Boolean"], ["Perceptual Rub & Buzz(phons)", "Boolean"], ["Measurement Confidence", "Boolean"], ["Total Diff", "Boolean"], ["THD(%)", "Boolean"], ["Standard Error", "Boolean"], ["Confidence Limits", "Boolean"], ["Total Noise", "Boolean"], ["Total IMD + Noise(%)", "Boolean"], ["Total DFD (%)", "Boolean"], ["Total IMD(%)", "Boolean"], ["Total IM", "Boolean"], ["Total DFD + Noise(%)", "Boolean"], ["+/-", "Numeric"], ["Orders IM", "List"], ["Orders Diff", "List"], ["Harmonics", "List"], ["Maxis", "Slide"], ["Delay Method", "Slide"], ["samples", "Numeric"], ["distance", "Numeric"], ["Applied Units", "Ring"], ["s", "Numeric"], ["CurveLibValues", "Boolean"], ["Record Delay", "Boolean"], ["TSR Window Type", "Ring"], ["Envelope?", "Boolean"], ["Result Waveforms", "Boolean"], ["Record Length (s)", "Numeric"], ["No.of FFTs", "Numeric"], ["Discard Cycles", "Numeric"], ["impulse resp?", "Boolean"], ["Start Time(s)", "Numeric"], ["StopTime(s)", "Numeric"], ["Scaling", "Ring"], ["Default Overlap", "Boolean"], ["Auto-Correlation(Stimulus)", "Boolean"], ["Auto-Correlation(Response)", "Boolean"], ["Deconvolved Response", "Boolean"], ["Weighting", "Ring"], ["Fmin(Hz)", "Numeric"], ["Fmax(Hz)", "Numeric"], ["Freq.Resolution(Hz)", "Numeric"], ["Over-samples Res.(Hz)", "Numeric"], ["Windowed Resolution(Hz)", "Numeric"], ["Overlap(%)", "Numeric"], ["Cross-Correlation", "Boolean"], ["Coupling", "Boolean"], ["AC/DC", "Slide"], ["Impedance", "Boolean"], ["Reference Resistor(ohm)", "Numeric"], ["DC Connect Measurement", "Boolean"], ["AC/DC 2", "Slide"], ["Use default", "Boolean"], ["Use Channel Name", "Boolean"], ["Custom Curve Names", "Table"], ["Unit", "String"], ["Type Out", "String"], ["Channel Out", "String"], ["Type in", "String"], ["Channel in", "String"], ["Waveforms In", "Ring"], ["Waveforms Out", "Ring"], ["Response Measurement", "Boolean"], ["Response", "Boolean"], ["Stimulus", "Boolean"], ["Response Measurement1", "Slide"], ["Apply Correction Out", "Boolean"], ["Apply Correction in", "Boolean"], ["Averaging", "Boolean"], ["Functions", "Boolean"], ["Spectral Scaling*", "Ring"], ["Auto-Spectrum(Stimulus)*", "Boolean"], ["Auto-Spectrum(Response)*", "Boolean"], ["Cross-Spectrum*", "Boolean"], ["Coherent Power*", "Boolean"], ["Frequency Response", "Boolean"], ["Non-Coherent Power*", "Boolean"], ["Coherence (%)", "Boolean"], ["Non-Coherence (%)", "Boolean"], ["Signal-Noise Ratio (dB)", "Boolean"], ["Non-Coherent Distortion*", "Boolean"], ["Averaging1", "Slide"], ["Loose Particle", "Boolean"], ["Loose Particle Waveform", "Boolean"], ["Averaging Time(s)", "Numeric"], ["Attack Threshold(dB)", "Numeric"], ["Max duration(s)", "Numeric"], ["Min duration(s)", "Numeric"], ["Hysteresis Up(dB)", "Numeric"], ["Apply", "Boolean"], ["units", "Boolean"], ["Edit List", "Boolean"], ["Main Tab", "Tab"], ["Advanced View", "Boolean"], ["Method", "Slide"], ["Coupling1", "Boolean"], ["Spectra", "Boolean"], ["Distance Unit", "Ring"], ["Curve Resolution", "Boolean"], ["Polarity", "Boolean"], ["Impedance Frame", "Boolean"], ["Amp Auto Mode", "Slide"], ["Mic Frame", "Boolean"], ["Mic Resistor(ohm)", "Numeric"], ["Mic Auto Mode", "Slide"], ["Mic Current", "Boolean"]], "Vi Ref"="Vi Ref") -> ()  [unwired: 9 in]
